vi "Chamber controller Dec 1 2016.vi"() -> ()   [LabVIEW 2014]
uses:
  <vilib>/Instr/_visa.llb/VISA Configure Serial Port (Instr).vi
  Environmental Chamber LabVIEW and Instruments/Drivers and Software/Keithley 2100 Series/Public/Configure/Configure 2 Wire Resistance.vi
  <vilib>/Utility/file.llb/Write To Spreadsheet File (string).vi
  <vilib>/Utility/file.llb/Read From Spreadsheet File (string).vi
  Environmental Chamber LabVIEW and Instruments/Drivers and Software/keithley_6430/Keithley 6430/Public/Data/Read (Single Point).vi
  Environmental Chamber LabVIEW and Instruments/Drivers and Software/LabVIEW 8.2 Drivers/keithley_24xx/Keithley 24XX/Public/Data/Read (Single Point).vi
  Environmental Chamber LabVIEW and Instruments/Drivers and Software/keithley_24xx/Keithley 24XX/Keithley 24XX.lvlib
  Environmental Chamber LabVIEW and Instruments/Drivers and Software/keithley_6430/Keithley 6430/Keithley 6430.lvlib
  Environmental Chamber LabVIEW and Instruments/Drivers and Software/Keithley 2100 Series/Keithley 2100 Series.lvlib
panel:
  in  "Arduino COMs":T1={"Arduino 1"="COM23", "Arduino 2"="COM24", "Arduino 3"="COM25", "Arduino 4"="COM26", "Arduino 5"="COM27", "Arduino 6"="COM28"}
  out "saving data?":bool
  out "ArduinoQCM\ncluster":T2 caption="Arduino QCM" {"6" format="%_8g"; "5" format="%_8g"; "4" format="%_8g"; "3" format="%_8g"; "2" format="%_8g"; "1" format="%#_10g"}
  in  "Data logging settings":T3={"Save during sequence only"=TRUE, "Save now"=FALSE, "sec between data points"=0.0, "Current data file path"=path "", "Save sample names"={"QCM1"="", "QCM2"="", "QCM3"="", "QCM4"="", "QCM5"="", "QCM6"="", "SRS"="", "K-2420"="", "K-6430"="", "K-2100"=""}, "Experiment Notes"=""} {"sec between data points" min=0.0 max=30.0 format="%#_13g"}
  in  "Sequence cluster":T4={"Save sequence"=FALSE, "Clear sequence"=FALSE, "Import sequence file"=FALSE, "Tare elapsed time"=TRUE, "Run Sequence"=FALSE, "Stop program when sequence ends"=TRUE, "User-defined\nsequence"=[], "Sequence end time"="", "Sequence\npreview"=[], "Current\nstep"=0, "Jump to next step"=FALSE} caption="Sequence settings"
  in  "Pressure parameters cluster":T5={"valve % open"=100.0, "Desired pressure"=0.0, "Vapor sccm"=0.0, "Gas sccm"=0.0, "Valve mode"=enum."% Open", "Pressure Mode"=enum."Abs. pressure", "analyte partial pressure"=23.8, "Turbo pump\nauto on"=TRUE, "Valve position (%)"=0.0, "read pressure"=0.0, "read vapor flow"=0.0, "read gas flow"=0.0, "pressure chart"={"pressure"=0.0}} caption="Pressure settings" {"read gas flow" format="%#_3g"; "read vapor flow" format="%#_3g"; "read pressure" format="%#_7f"; "Valve position (%)" format="%#_3g"; "analyte partial pressure" min=0.0 max=100.0 step=5.0; "Gas sccm" min=0 max=200 step=5; "Vapor sccm" min=0 max=200 step=5; "Desired pressure" min=0.0 max=760.0 step=5.0; "valve % open" min=0.0 max=100.0 step=5.0 format="%#_2f"}
  out "J-KEM temp chart":dbl(graph)
  out "Elapsed time (min)":dbl
  out "State date/time":string caption="Start time"
  out "K-2100 (Ohm)":cluster{"Measurement":dbl}(graph) caption="K-2100"
  out "K-6430":cluster{"Measurement":dbl}(graph)
  out "K-2420":cluster{"Resistance":sgl}(graph)
  in  "Gate time (sec)":enum16{"0.1", "1.0 ", "10"}(ring)=enum."1.0 "
  out "Hz":dbl format="%.7f"
  out "QCM plot":T6(graph)
  in  "Stop":bool
  in  "Clear all charts":bool
  out "O2 sensor output":dbl[](array[numeric]) caption="atm\nTorr"
  in  "rapidox O2 Sensor":bool
  in  "setnag O2 Pump":bool
  in  "Baud Rate 2":i32(ring)=2 items=["2400", "4800", "9600", "19200", "38400", "57600", "115200"]
  in  "Com Port":i32(ring) items=["Com 1", "Com 2", "Com 3", "Com 4", "Com 5", "Com 6", "COM 7", "COM 8", "COM 9", "COM 10", "COM 11", "COM 12", "com 13", "COM 14"]
  in  "Com Port 2":i32(ring) items=["Com 1", "Com 2", "Com 3", "Com 4", "Com 5", "Com 6", "COM 7", "COM 8", "COM 9", "COM 10", "COM 11", "COM 12", "com 13", "COM 14"]
  out "Waveform Chart":cluster{dbl}(graph)
  out "O2 Concentration (PPM)":dbl
  out "Waveform Chart 6":cluster{dbl}(graph)
  # "Currently Unused"
  # "100%"
  # "SRS"
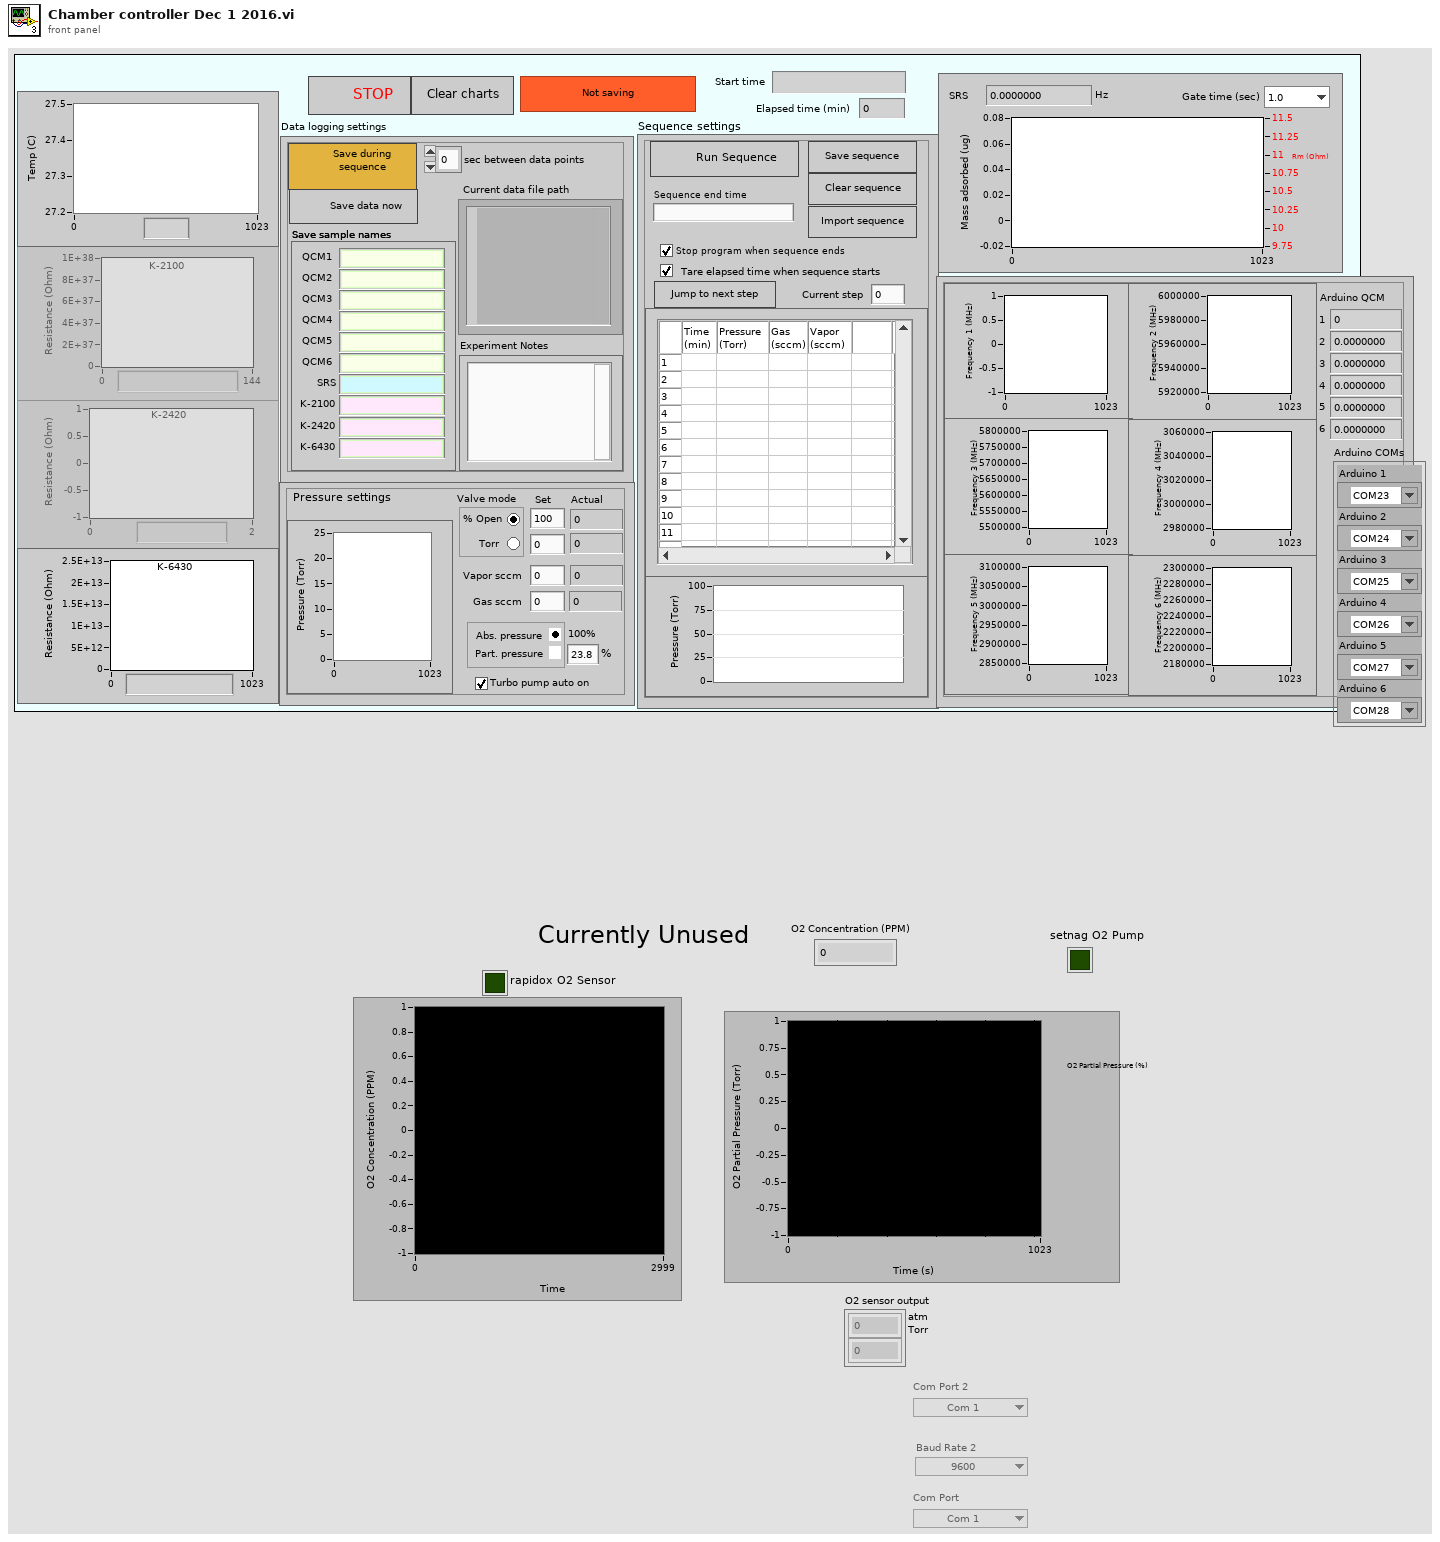
[diagram p1: front panel]
types:
  T1 = cluster{"Arduino 1":refnum<visa-resource-name>, "Arduino 2":refnum<visa-resource-name>, "Arduino 3":refnum<visa-resource-name>, "Arduino 4":refnum<visa-resource-name>, "Arduino 5":refnum<visa-resource-name>, "Arduino 6":refnum<visa-resource-name>}
  T2 = cluster{"arduino qcm 1":dbl, "1":dbl, "arduino qcm 2":dbl, "2":dbl, "arduino qcm 3":dbl, "3":dbl, "arduino qcm 4":dbl, "4":dbl, "arduino qcm 5":dbl, "5":dbl, "arduino qcm 6":dbl, "6":dbl}
  T3 = cluster{"Save during sequence only":bool, "Save now":bool, "sec between data points":dbl, "Current data file path":path, "Save sample names":cluster{"QCM1":string, "QCM2":string, "QCM3":string, "QCM4":string, "QCM5":string, "QCM6":string, "SRS":string, "K-2420":string, "K-6430":string, "K-2100":string}, "Experiment Notes":string}
  T4 = cluster{"Save sequence":bool, "Clear sequence":bool, "Import sequence file":bool, "Tare elapsed time":bool, "Run Sequence":bool, "Stop program when sequence ends":bool, "User-defined\nsequence":string[][], "Sequence end time":string, "Sequence\npreview":cluster{dbl[], dbl[]}[], "Current\nstep":i32, "Jump to next step":bool}
  T5 = cluster{"valve % open":dbl, "Desired pressure":dbl, "Vapor sccm":sgl, "Gas sccm":sgl, "Valve mode":enum32{"% Open", "Torr "}, "Pressure Mode":enum32{"Abs. pressure", " Part. pressure"}, "analyte partial pressure":dbl, "Turbo pump\nauto on":bool, "Valve position (%)":dbl, "read pressure":dbl, "read vapor flow":dbl, "read gas flow":dbl, "pressure chart":cluster{"pressure":dbl}}
  T6 = cluster{"Numeric Control":dbl, "Resistance out":dbl}
  T7 = cluster{"Keithley 6430":bool, "J-KEM":bool, "Keithley 2420":bool, "Keithley 2100":bool, "SRS QCM":bool, "Pressure control":bool, "Arduino":bool}
  T8 = enum8{"Enabled", "Disabled", "Disabled and Grayed Out"}
  T9 = enum16{"open", "open or create", "create or replace", "create", "open (read only)"}
  T10 = enum16{"no parity", "odd parity", "even parity", "mark parity", "space parity"}
  T11 = cluster{"String":string, "String":string, "String":string}
  T12 = cluster{"task out":refnum<k21>, "error out":errorcluster, "task out":refnum<k21>, "error out":errorcluster, "task out":refnum<k21>, "error out":errorcluster, "VISA resource name":refnum<visa-resource-name>, "error out":errorcluster}
  T13 = cluster{"task out":refnum<k21>, "error out":errorcluster, "task out":refnum<k21>, "error out":errorcluster, "task out":refnum<k21>, "error out":errorcluster, "VISA resource name out":refnum<visa-resource-name>, "error out":errorcluster}
  T14 = cluster{bool, "VISA resource name":refnum<visa-resource-name>, "error out":errorcluster}
  T15 = cluster{bool, "VISA resource name out":refnum<visa-resource-name>, "error out":errorcluster}
  T16 = cluster{"VISA resource name out":refnum<visa-resource-name>, "error out":errorcluster, "VISA resource name out":refnum<visa-resource-name>, "error out":errorcluster, "VISA resource name out":refnum<visa-resource-name>, "error out":errorcluster, "VISA resource name out":refnum<visa-resource-name>, "error out":errorcluster, "VISA resource name out":refnum<visa-resource-name>, "error out":errorcluster, "VISA resource name out 2":refnum<visa-resource-name>, "error out 2":errorcluster}
  T17 = cluster{bool, cluster{"task out":refnum<k21>, "error out":errorcluster, "task out":refnum<k21>, "error out":errorcluster, "task out":refnum<k21>, "error out":errorcluster, "VISA resource name out":refnum<visa-resource-name>, "error out":errorcluster}}
  T18 = cluster{"f":dbl, "f":dbl, "f":dbl, "f":dbl, "f":dbl, "f 2":dbl}
  T19 = cluster{"Boolean":bool, "VISA resource name out":refnum<visa-resource-name>, "error out":errorcluster}
  T20 = cluster{bool, "VISA out":refnum<visa-resource-name>, "error out":errorcluster}
  T21 = cluster{"Boolean":bool, "VISA out":refnum<visa-resource-name>, "error out":errorcluster}
  T22 = cluster{"Numeric Control":dbl, "Cluster":cluster{"Numeric Control":dbl}, "String":string, "error out":errorcluster}
  T23 = cluster{bool, "Com Port":i32, "Numeric Control out":dbl}
  T24 = cluster{"Arduino address":refnum<visa-resource-name>, "error in (no error)":errorcluster, "Arduino address 2":refnum<visa-resource-name>, "error in (no error) 2":errorcluster, "Arduino address 3":refnum<visa-resource-name>, "error in (no error) 3":errorcluster, "Arduino address 4":refnum<visa-resource-name>, "error in (no error) 4":errorcluster, "Arduino address 5":refnum<visa-resource-name>, "error in (no error) 5":errorcluster, "Arduino address 6":refnum<visa-resource-name>, "error in (no error) 6":errorcluster}
  T25 = cluster{"mean":string, "mean":string, "mean":string, "mean":string, "mean":string, "mean":string}
  T26 = cluster{"String data out":string, string, string, string}
  T27 = cluster{"valve % open":dbl, "Desired pressure":dbl, "Vapor sccm":sgl, "Gas sccm":sgl, "Valve mode":enum32{"% Open", "Torr "}, "Pressure Mode":enum32{"Abs. pressure", " Part. pressure"}, "analyte partial pressure":dbl, "Turbo pump\nauto on":bool}
  T28 = cluster{"User-defined\nsequence":string[][], "Present (s)":dbl, "current  step # in":i32, "sequence end time in":timestamp}
  T29 = cluster{"current  step # in":i32, "sequence end time in":timestamp, "Boolean":bool}
  T30 = cluster{"press/RH/gas/vapor":cluster{"pressure":string, "RH":string, "gas flow":string, "vapor flow":string}, "Cluster":cluster{"Valve position (%)":dbl, "read pressure":dbl, "read vapor flow":dbl, "read gas flow":dbl}}
  T31 = cluster{"Boolean":bool, "DAQ IDs in":cluster{"task out":refnum<k21>, "error out":errorcluster, "task out":refnum<k21>, "error out":errorcluster, "task out":refnum<k21>, "error out":errorcluster, "VISA Refnum out":refnum<visa-resource-name>, "error out":errorcluster}}
  T32 = cluster{"mean":dbl, "mean":dbl, "mean":dbl, "mean":dbl, "mean":dbl, "mean":dbl}
  T33 = cluster{"f":dbl, "f":dbl, "f":dbl, "f":dbl, "f":dbl}[]
  T34 = cluster{"pressure":string, "RH":string, "gas flow":string, "vapor flow":string}
  T35 = cluster{"Valve position (%)":dbl, "read pressure":dbl, "read vapor flow":dbl, "read gas flow":dbl}
  T36 = cluster{"mean":dbl, "mean":dbl, "mean":dbl, "mean":dbl, "mean":dbl, "mean":dbl, "mean":dbl, "mean":dbl, "mean":dbl, "mean":dbl, "mean":dbl, "mean":dbl}
  T37 = cluster{"QCM1":string, "QCM2":string, "QCM3":string, "QCM4":string, "QCM5":string, "QCM6":string, "SRS":string, "K-2420":string, "K-6430":string, "K-2100":string}
  T38 = cluster{"task out":refnum<k21>, "error out":errorcluster, "task out":refnum<k21>, "error out":errorcluster, "task out":refnum<k21>, "error out":errorcluster, "VISA Refnum out":refnum<visa-resource-name>, "error out":errorcluster}
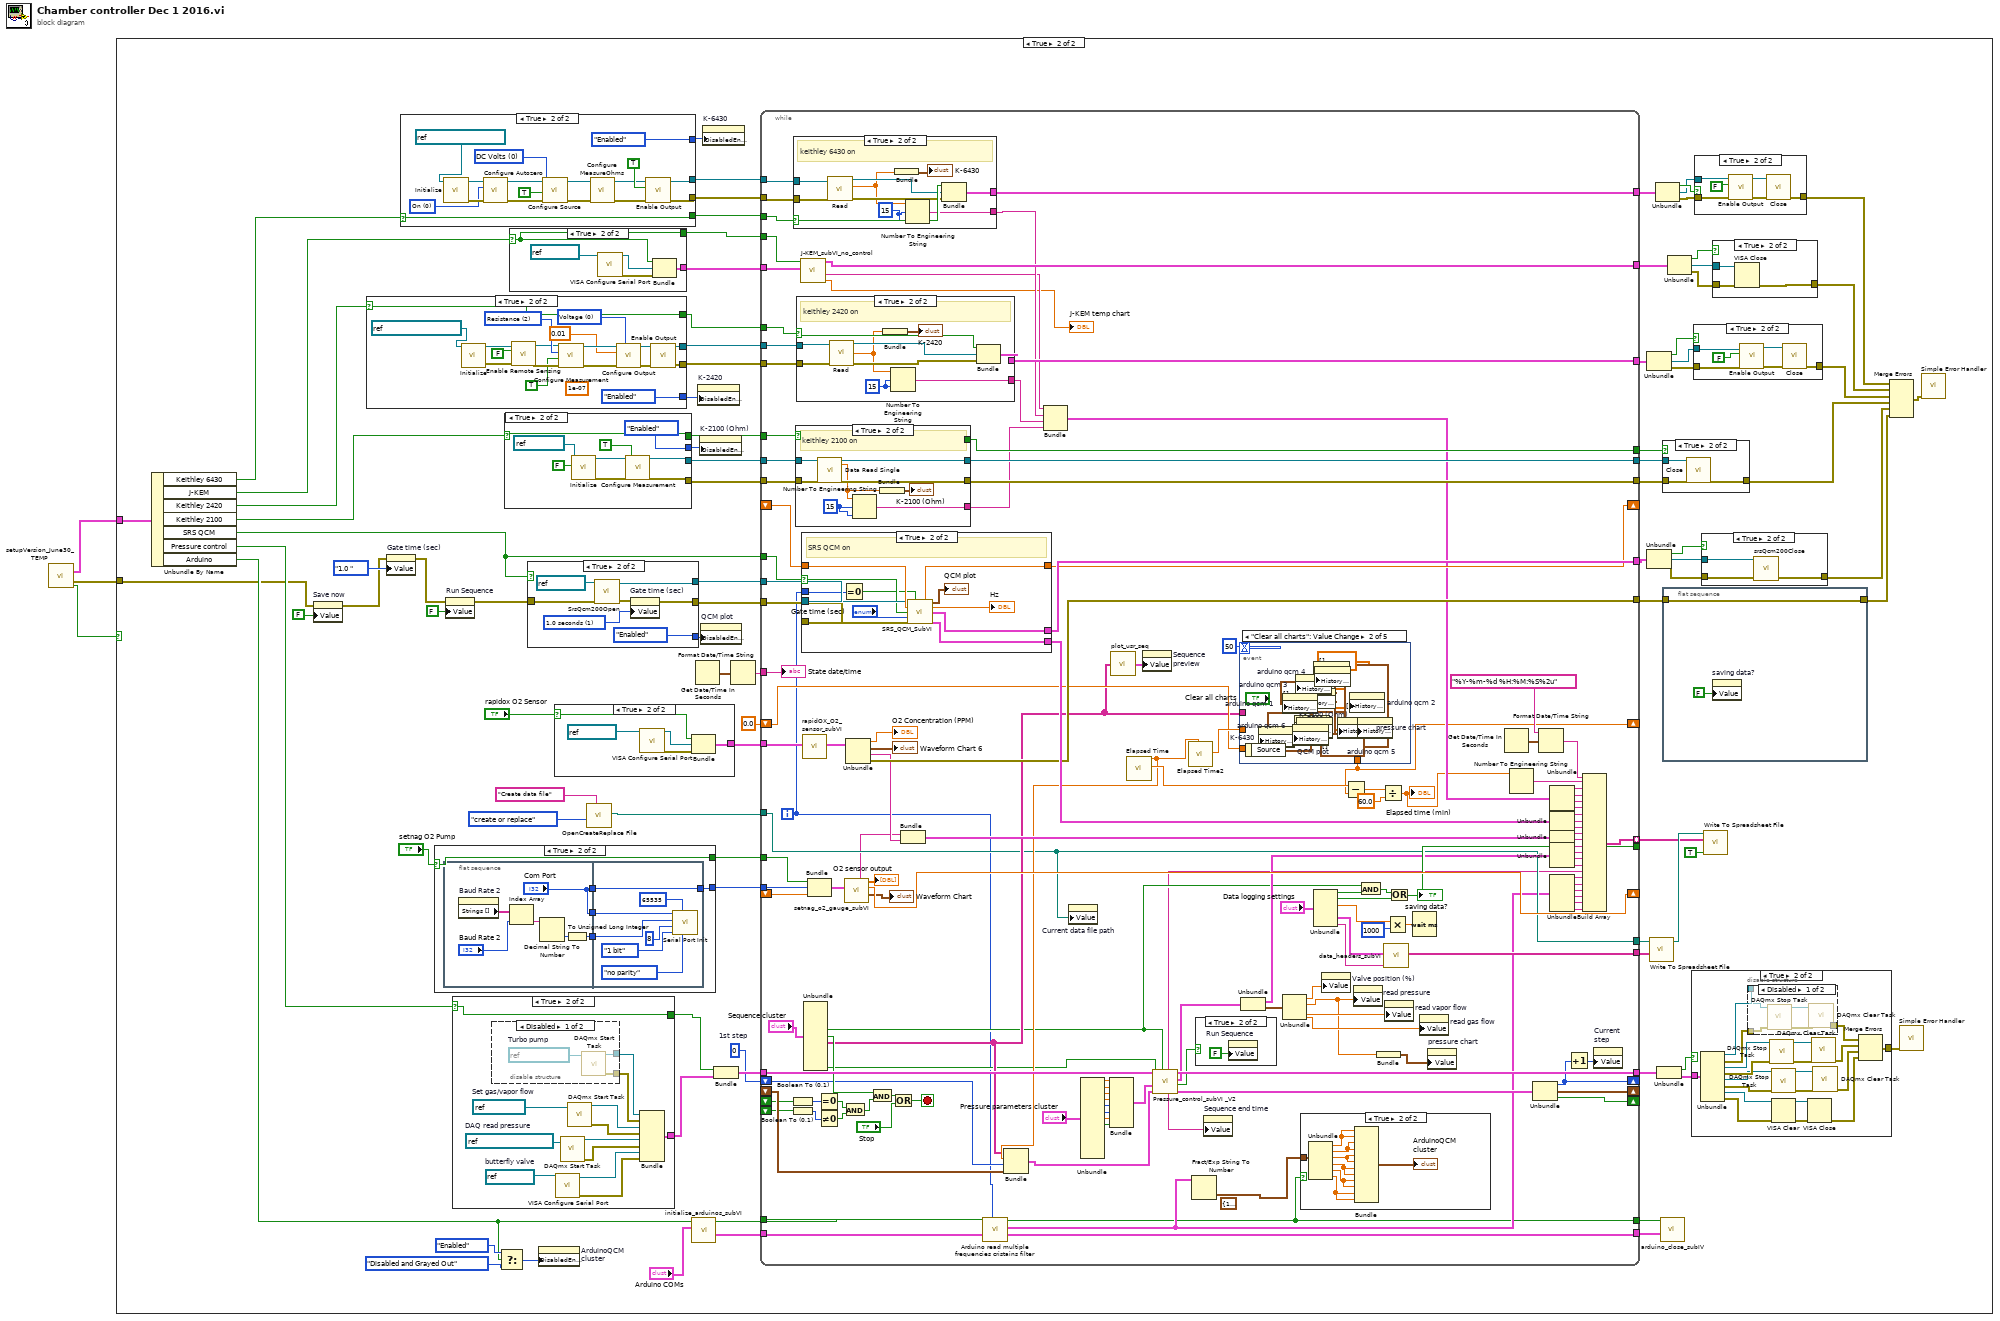
[diagram p0: block diagram]
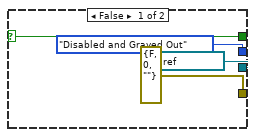
[diagram p4: hidden frame]
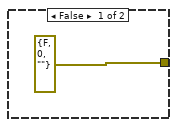
[diagram p5: hidden frame]
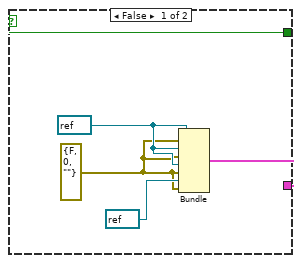
[diagram p7: hidden frame]
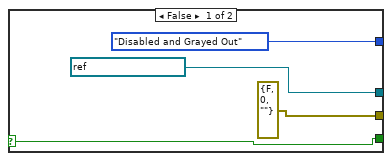
[diagram p10: hidden frame]
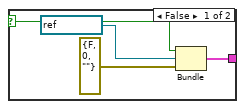
[diagram p11: hidden frame]
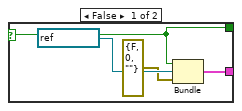
[diagram p13: hidden frame]
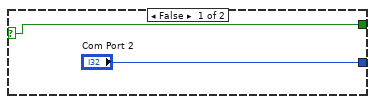
[diagram p14: hidden frame]
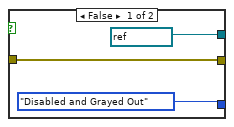
[diagram p16: hidden frame]
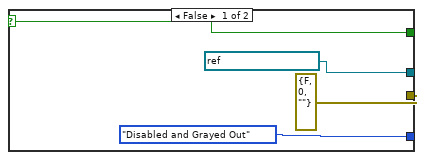
[diagram p18: hidden frame]
diagram:
  n1 = call "setupVersion_June30_TEMP.vi"() -> ("Instruments on/off"=w1:T7, "error IO"=w2:errorcluster, "OK"=w3:bool)  [unwired: 13 in]
  n2 = case shown="True" w3 {
    tunnel: w2 -> [_ w8]
    tunnel: w1 -> [_ w16]
    frame False {
    }
    frame True {
      w28 = 0  # 1st step
      n3 = Unbundle By Name(w16) -> ("Keithley 6430"=w15:bool, "J-KEM"=w14:bool, "Keithley 2420"=w13:bool, "Keithley 2100"=w12:bool, "SRS QCM"=w11:bool, "Pressure control"=w10:bool, "Arduino"=w9:bool)
      n4 = property on="Save now" class="Bool (strict)"(error in=w8, "Value"=FALSE) -> (error out=w7:errorcluster)  [unwired: 1 in, 1 out]
      n5 = case shown="True" w13 {
        selector: w13 -> [w252 w256]
        tunnel: [refnum<visa-resource-name> "GPIB1::24::INSTR" ("VISA resource name") w265] -> w92
        tunnel: [errorcluster {"status"=FALSE, "code"=0, "source"=""} ("error out") w260] -> w91
        tunnel: [T8."Disabled and Grayed Out" ("Disabled") T8."Enabled" ("Disabled")] -> w55
        tunnel: [w252 w256] -> w48
        frame False {
        }
        frame True {
          (unwired) 1e-07 ("Manual Range (1.0)")
          w267 = u16 0 items=["Voltage", "Current"] ("Source Mode  (0: Voltage)")
          w272 = u16 2 items=["Volts", "Current", "Resistance"] ("Function (0: Volts)")
          n6 = call "Initialize.vi"("VISA resource name"=refnum<visa-resource-name> "GPIB1::24::INSTR") -> ("error out"=w261:errorcluster, "VISA resource name out"=w264:refnum<visa-resource-name>)  [unwired: 9 in]
          n7 = call "Enable Remote Sensing.vi"("error in (no error)"=w261, "Enable Remote Sensing (T: Enable)"=FALSE ("4-wire?"), "VISA resource name"=w264) -> ("error out"=w262:errorcluster, "VISA resource name out"=w263:refnum<visa-resource-name>)  [unwired: 7 in]
          n8 = call "Configure Measurement.vi"("error in (no error)"=w262, "Enable Auto Range (T:Enable)"=TRUE, "Function (0: Volts)"=w272, "VISA resource name"=w263) -> ("error out"=w271:errorcluster, "VISA resource name out"=w270:refnum<visa-resource-name>)  [unwired: 6 in]
          n9 = call "Configure Output.vi"("Source Mode  (0: Voltage)"=w267, "error in (no error)"=w271, "Output Level (0)"=0.01 ("Applied Voltage (V)"), "VISA resource name"=w270) -> ("error out"=w269:errorcluster, "VISA resource name out"=w268:refnum<visa-resource-name>)  [unwired: 6 in]
          n10 = call "Enable Output.vi"("error in (no error)"=w269, "VISA resource name"=w268) -> ("error out"=w260:errorcluster, "VISA resource name out"=w265:refnum<visa-resource-name>)  [unwired: 8 in]
        }
      }
      n11 = property on="Gate time (sec)" class="Enum (strict)"(error in=w7, "Value"=enum16{"0.1", "1.0 ", "10"}."1.0 " ("Gate time (sec)")) -> (error out=w17:errorcluster)  [unwired: 1 in, 1 out]
      n12 = case shown="True" w15 {
        selector: w15 -> [w168 w172]
        tunnel: [refnum<visa-resource-name> "GPIB0::29::INSTR" ("VISA resource name") w183] -> w61
        tunnel: [errorcluster {"status"=FALSE, "code"=0, "source"=""} ("error out") w184] -> w60
        tunnel: [T8."Disabled and Grayed Out" ("Disabled") T8."Enabled" ("Disabled")] -> w54
        tunnel: [w168 w172] -> w47
        frame False {
        }
        frame True {
          w173 = u16 0 items=["DC Volts", "DC Current"] ("Source Function (0: DC Volts)")
          w180 = u16 0 items=["On", "Off", "Once"] ("Autozero  (0: On)")
          n13 = call "Initialize.vi"("VISA resource name"=refnum<visa-resource-name> "GPIB0::29::INSTR") -> ("error out"=w181:errorcluster, "VISA resource name out"=w182:refnum<visa-resource-name>)  [unwired: 4 in, 5 out]
          n14 = call "Configure Autozero.vi"("error in (no error)"=w181, "Autozero  (0: On)"=w180, "VISA resource name"=w182) -> ("error out"=w176:errorcluster, "VISA resource name out"=w178:refnum<visa-resource-name>)  [unwired: 7 in]
          n15 = call "Configure Source.vi"("error in (no error)"=w176, "Auto Range (T:Enable)"=TRUE, "Source Function (0: DC Volts)"=w173, "VISA resource name"=w178) -> ("error out"=w175:errorcluster, "VISA resource name out"=w177:refnum<visa-resource-name>)  [unwired: 6 in]
          n16 = call "Configure MeasureOhms.vi"("error in (no error)"=w175, "VISA resource name"=w177) -> ("error out"=w188:errorcluster, "VISA resource name out"=w186:refnum<visa-resource-name>)  [unwired: 4 in, 4 out]
          n17 = call "Enable Output.vi"("error in (no error)"=w188, "Enable Output (F:Off)"=TRUE ("Output (F:Off)"), "VISA resource name"=w186) -> ("error out"=w184:errorcluster, "VISA resource name out"=w183:refnum<visa-resource-name>)  [unwired: 7 out]
        }
      }
      n18 = case shown="True" "setnag O2 Pump" {
        selector: "setnag O2 Pump" -> [w211 w213]
        tunnel: ["Com Port 2" w214] -> w88
        tunnel: [w211 w213] -> w36
        frame False {
        }
        frame True {
          n19 = flat-sequence {
            tunnel: ["Com Port"] -> w217
            tunnel: [w219] -> w216
            tunnel: ["Com Port"] -> w215
            tunnel: w217 -> [w225]
            tunnel: w216 -> [w224]
            tunnel: w215 -> [w226]
            tunnel: [w226] -> w214
            frame #0 {
              n20 = property on="Baud Rate 2" class="Ring (strict)"() -> ("Strings []"=w221:string[])  [unwired: 2 in, 2 out]
              n21 = Index Array(array=w221, index="Baud Rate 2") -> (element=w222:string)
              n22 = Decimal String To Number(string=w222) -> (number=w220:i32)  [unwired: 2 in, 1 out]
              n23 = To Unsigned Long Integer(number=w220) -> (unsigned 32bit integer=w219:u32)
            }
            frame #1 {
              n24 = call <vilib>:"Serial Port Init.vi"("parity"=T10."no parity", "buffer size"=u16 65535, "stop bits"=enum16{"1 bit", "1.5 bits", "2 bits"}."1 bit", "data bits"=u16 8, "baud rate"=w224, "port number"=w225) -> ()  [unwired: 1 in, 1 out]
            }
          }
        }
      }
      n25 = property on="Run Sequence" class="Bool (strict)"(error in=w17, "Value"=FALSE) -> (error out=w23:errorcluster)  [unwired: 1 in, 1 out]
      n26 = case shown="True" w10 {
        selector: w10 -> [w140 w145]
        tunnel: [w141 w147] -> w30
        tunnel: [w140 w145] -> w31
        frame False {
          w143 = refnum<k21> refnum ("task out")
          w142 = errorcluster {"status"=FALSE, "code"=0, "source"=""} ("error out")
          n27 = Bundle("task out"=w143, "error out"=w142, "task out"=w143, "error out"=w142, "task out"=w143, "error out"=w142, "VISA resource name"=refnum<visa-resource-name> refnum, "error out"=w142) -> (w141:T12)  [unwired: 1 in]
        }
        frame True {
          w155 = refnum<visa-resource-name> "COM5"  # butterfly valve
          w156 = refnum<k21> "Setflow"  # Set gas/vapor flow
          w157 = refnum<k21> "AllDaqReadings"  # DAQ read pressure
          n28 = disable-structure shown="Disabled" {
            disable-tunnel: [w159 _] -> w154
            disable-tunnel: [w158 _] -> w153
            frame Disabled {
              w160 = refnum<k21> "TurboON"  # Turbo pump
              n29 = call <vilib>:"DAQmx Start Task.vi"("task/channels in"=w160) -> ("task out"=w159:refnum<k21>, "error out"=w158:errorcluster)  [unwired: 13 in]
            }
            frame Enabled {
            }
          }
          n30 = call-poly "VISA Configure Serial Port"("VISA resource name"=w155) -> ("VISA resource name out"=w148:refnum<visa-resource-name>, "error out"=w146:errorcluster)  [unwired: 13 in]
          n31 = call <vilib>:"DAQmx Start Task.vi"("task/channels in"=w157) -> ("task out"=w150:refnum<k21>, "error out"=w149:errorcluster)  [unwired: 13 in]
          n32 = call <vilib>:"DAQmx Start Task.vi"("task/channels in"=w156) -> ("task out"=w152:refnum<k21>, "error out"=w151:errorcluster)  [unwired: 13 in]
          n33 = Bundle("task out"=w154, "error out"=w153, "task out"=w152, "error out"=w151, "task out"=w150, "error out"=w149, "VISA resource name out"=w148, "error out"=w146) -> (w147:T13)  [unwired: 1 in]
        }
      }
      n34 = Select(t=T8."Enabled" ("Disabled"), s=w9, f=T8."Disabled and Grayed Out" ("Disabled")) -> (s? t:f=w22:T8)
      n35 = case shown="True" w12 {
        selector: w12 -> [w102 w107]
        tunnel: [refnum<visa-resource-name> "K-2100" ("VISA resource name out") w110] -> w45
        tunnel: [errorcluster {"status"=FALSE, "code"=0, "source"=""} ("error out") w109] -> w44
        tunnel: [w102 w107] -> w43
        tunnel: [T8."Disabled and Grayed Out" ("Disabled") T8."Enabled" ("Disabled")] -> w38
        frame False {
        }
        frame True {
          n36 = call "Initialize.vi"("VISA resource name"=refnum<visa-resource-name> "K-2100", "Reset? (T: Reset)"=FALSE) -> ("VISA resource name out"=w111:refnum<visa-resource-name>, "error out"=w108:errorcluster)  [unwired: 16 in]
          n37 = call-poly "Configure Measurement.vi"("VISA resource name"=w111, "error in (no error)"=w108, "Auto Range? (T: Auto)"=TRUE) -> ("VISA resource name out"=w110:refnum<visa-resource-name>, "error out"=w109:errorcluster)  [unwired: 15 in]
        }
      }
      n38 = case shown="True" w14 {
        selector: w14 -> [w202 w207]
        tunnel: [w203 w208] -> w77
        tunnel: [w202 w207] -> w71
        frame False {
          n39 = Bundle(w202, "VISA resource name"=refnum<visa-resource-name> "COM3", "error out"=errorcluster {"status"=FALSE, "code"=0, "source"=""}) -> (w203:T14)  [unwired: 1 in]
        }
        frame True {
          n40 = call-poly "VISA Configure Serial Port"("VISA resource name"=refnum<visa-resource-name> "COM3") -> ("VISA resource name out"=w209:refnum<visa-resource-name>, "error out"=w206:errorcluster)  [unwired: 13 in]
          n41 = Bundle(w207, "VISA resource name out"=w209, "error out"=w206) -> (w208:T15)  [unwired: 1 in]
        }
      }
      n42 = case shown="True" w11 {
        tunnel: [refnum<visa-resource-name> "COM6" ("VISA in") w241] -> w90
        tunnel: [w236 w238] -> w89
        tunnel: w23 -> [w236 w243]
        tunnel: [T8."Disabled and Grayed Out" ("Disabled") T8."Enabled" ("Disabled")] -> w56
        frame False {
        }
        frame True {
          w240 = u16 1 items=["0.1 seconds", "1.0 seconds", "10.0 seconds"] ("Gate time")
          n43 = call "SrsQcm200Open.vi"("error in"=w243, "VISA in"=refnum<visa-resource-name> "COM6") -> ("error out"=w239:errorcluster, "VISA out"=w241:refnum<visa-resource-name>)  [unwired: 3 in]
          n44 = property on="Gate time (sec)" class="Enum (strict)"(error in=w239, "Value"=w240) -> (error out=w238:errorcluster)  [unwired: 1 in, 1 out]
        }
      }
      n45 = property on="ArduinoQCM\ncluster" class="Clust (strict)"("DisabledEnum"=w22) -> ()  [unwired: 2 in, 2 out]
      n46 = case shown="True" "rapidox O2 Sensor" {
        selector: "rapidox O2 Sensor" -> [w189 w194]
        tunnel: [w190 w195] -> w67
        frame False {
          n47 = Bundle(w189, "VISA resource name"=refnum<visa-resource-name> "COM7", "error out"=errorcluster {"status"=FALSE, "code"=0, "source"=""}) -> (w190:T14)  [unwired: 1 in]
        }
        frame True {
          n48 = call-poly "VISA Configure Serial Port"("VISA resource name"=refnum<visa-resource-name> "COM7") -> ("VISA resource name out"=w196:refnum<visa-resource-name>, "error out"=w193:errorcluster)  [unwired: 13 in]
          n49 = Bundle(w194, "VISA resource name out"=w196, "error out"=w193) -> (w195:T15)  [unwired: 1 in]
        }
      }
      n50 = call "OpenCreateReplace File.vi"("prompt"="Create data file", "function (open:0)"=T9."create or replace") -> ("new file path"=w46:path)  [unwired: 6 in, 3 out]
      n51 = call "initialize_arduinos_subVI.vi"("arduino 1-6 addresses"="Arduino COMs", "arduinos on?"=w9) -> ("arduino addresses/errors"=w32:T16, "arduinos on/off"=w52:bool)  [unwired: 8 in]
      n52 = Get Date/Time In Seconds() -> (seconds since 1Jan1904=w94:timestamp)
      n53 = property on="K-2420" class="WFChart (strict)"("DisabledEnum"=w55) -> ()  [unwired: 2 in, 2 out]
      n54 = property on="K-2100 (Ohm)" class="WFChart (strict)"("DisabledEnum"=w38) -> ()  [unwired: 2 in, 2 out]
      n55 = property on="QCM plot" class="WFChart (strict)"("DisabledEnum"=w56) -> ()  [unwired: 2 in, 2 out]
      n56 = property on="K-6430" class="WFChart (strict)"("DisabledEnum"=w54) -> ()  [unwired: 2 in, 2 out]
      n57 = Bundle(w31, w30) -> (w29:T17)  [unwired: 1 in]
      n58 = Format Date/Time String(seconds (now)=w94) -> (date/time string=w35:string)  [unwired: 2 in]
      n59 = while {
        shift-right: [w417] -> _
        shift-left: _ -> [w348]
        tunnel: [w401] -> w53 mode=indexing if=w370
        tunnel: w48 -> [w406]
        tunnel: w92 -> [w416]
        tunnel: w91 -> [w415]
        tunnel: w90 -> [w414]
        tunnel: w89 -> [w413]
        tunnel: w11 -> [w412]
        tunnel: w36 -> [w350]
        tunnel: w88 -> [w351]
        tunnel: [w411] -> w85
        tunnel: [w410] -> w81
        tunnel: w77 -> [w409]
        tunnel: [w408] -> w76
        tunnel: w71 -> [w407]
        tunnel: w67 -> [w359]
        tunnel: [w355] -> w5
        tunnel: [w290] -> w66
        tunnel: w46 -> [w290]
        shift-right: [w399] -> _
        shift-left: _ -> [w400]
        tunnel: w61 -> [w405]
        tunnel: w60 -> [w404]
        tunnel: [w403] -> w59
        tunnel: [w370] -> _
        tunnel: w52 -> [w277]
        tunnel: w32 -> [w280]
        tunnel: [w276] -> w50
        tunnel: [w278] -> w51
        tunnel: [w387] -> w49
        tunnel: w47 -> [w382]
        tunnel: w45 -> [w369]
        tunnel: w44 -> [w368]
        tunnel: w43 -> [w367]
        tunnel: [w366] -> w42
        tunnel: [w365] -> w41
        tunnel: [w364] -> w40
        shift-right: [w342] -> _
        shift-left: 0.0 ("Elapsed Time (s)") -> [w343]
        tunnel: w35 -> [w333]
        tunnel: w29 -> [w315]
        shift-right: [w285] -> _
        shift-left: w28 -> [w304]
        shift-right: [w310] -> _
        shift-left: _ -> [w308]
        shift-right: [w309] -> _
        shift-left: _ -> [w307]
        shift-left: _ -> [w306]
        tunnel: [w302] -> w27
        i -> [w275]
        stop <- w372 stop-if-true
        (unwired) T18 {"f"=1000000.0, "f"=1000000.0, "f"=1000000.0, "f"=1000000.0, "f"=1000000.0, "f 2"=1000000.0} ("y")
        n60 = Boolean To (0,1)(Boolean=w307) -> (0, 1=w380:i16)
        n61 = Boolean To (0,1)(Boolean=w306) -> (0, 1=w379:i16)
        n62 = case "Keithley 6430" shown="True" w382 {
          selector: w382 -> [w452 w463]
          tunnel: w405 -> [w451 w460]
          tunnel: w404 -> [w450 w459]
          tunnel: ["" w462] -> w354
          tunnel: [w449 w461] -> w403
          frame False {
            # "keithley 6430 off"
            n63 = Bundle(w452, "VISA resource name out"=w451, "error out"=w450) -> (w449:T15)  [unwired: 1 in]
          }
          frame True {
            w454 = i16 15 ("width (-)")
            # "keithley 6430 on"
            n64 = call-poly "Read.vi"("error in (no error)"=w459, "VISA resource name"=w460) -> ("error out"=w458:errorcluster, "Measurement"=w456:dbl, "VISA resource name out"=w457:refnum<visa-resource-name>)  [unwired: 1 in, 6 out]
            n65 = Bundle("Measurement"=w456) -> (→"K-6430":cluster{"Measurement":dbl})  [unwired: 1 in]
            n66 = Number To Engineering String(2:w454, 3:w454, 4:w456) -> (0:w462:string)  [unwired: 1 in]
            n67 = Bundle(w463, "VISA resource name out"=w457, "error out"=w458) -> (w461:T15)  [unwired: 1 in]
          }
        }
        n68 = case shown="True" w367 {
          selector: w367 -> [w428 w433]
          tunnel: [w429 w440] -> w365
          tunnel: [w430 w439] -> w364
          tunnel: w369 -> [w429 w438]
          tunnel: w368 -> [w430 w437]
          tunnel: ["" w435] -> w352
          tunnel: [w428 w433] -> w366
          frame False {
            # "keithley 2100 off"
          }
          frame True {
            w432 = i16 15 ("width (-)")
            # "keithley 2100 on"
            n69 = call "Data Read Single.vi"("VISA resource name"=w438, "error in (no error)"=w437) -> ("VISA resource name out"=w440:refnum<visa-resource-name>, "Measurement"=w436:dbl, "error out"=w439:errorcluster)  [unwired: 15 in]
            n70 = Number To Engineering String ("elapsed time (min)")(2:w432, 3:w432, 4:w436) -> (0:w435:string)  [unwired: 1 in]
            n71 = Bundle("Measurement"=w436) -> (→"K-2100 (Ohm)":cluster{"Measurement":dbl})  [unwired: 1 in]
          }
        }
        n72 = case "Keithley 2420" shown="True" w406 {
          selector: w406 -> [w467 w476]
          tunnel: w416 -> [w466 w471]
          tunnel: w415 -> [w465 w470]
          tunnel: [w464 w474] -> w411
          tunnel: ["" w473] -> w353
          frame False {
            # "keithley 2420 off"
            n73 = Bundle(w467, "VISA resource name out"=w466, "error out"=w465) -> (w464:T15)  [unwired: 1 in]
          }
          frame True {
            w469 = i16 15 ("width (-)")
            # "keithley 2420 on"
            n74 = call-poly "Read.vi"("VISA resource name"=w471, "error in (no error)"=w470) -> ("VISA resource name out"=w477:refnum<visa-resource-name>, "Resistance"=w472:sgl, "error out"=w475:errorcluster)  [unwired: 7 in, 4 out]
            n75 = Bundle("Resistance"=w472) -> (→"K-2420":cluster{"Resistance":sgl})  [unwired: 1 in]
            n76 = Number To Engineering String(2:w469, 3:w469, 4:w472) -> (0:w473:string)  [unwired: 1 in]
            n77 = Bundle(w476, "VISA resource name out"=w477, "error out"=w475) -> (w474:T15)  [unwired: 1 in]
          }
        }
        n78 = call "J-KEM_subVI_no_control.vi"("Address in"=w409, "J-KEM on?"=w407) -> ("Temp (C)"=→"J-KEM temp chart":dbl, "String data out"=w341:string, "Address out"=w408:T19)  [unwired: 6 in, 1 out]
        n79 = case "SRS QCM" shown="True" w412 {
          selector: w412 -> [w481 w490]
          tunnel: w414 -> [w484 w492]
          tunnel: w413 -> [w483 w493]
          tunnel: [w482 w496] -> w410
          tunnel: w400 -> [w479 w495]
          tunnel: [w479 w494] -> w399
          tunnel: [T11 {"String"="", "String"="", "String"=""} ("M,F,MR output cluster") w489] -> w392
          tunnel: w275 -> [_ w486]
          frame False {
            # "SRS QCM off"
            n80 = Bundle(w481, "VISA out"=w484, "error out"=w483) -> (w482:T20)  [unwired: 1 in]
          }
          frame True {
            # "SRS QCM on"
            n81 = Equal To 0?(x=w486) -> (x = 0?=w487:bool)
            n82 = call "SRS_QCM_SubVI.vi"("VISA Refnum in"=w492, "first iteration?"=w487, "Frequency out 3"=w495, "Boolean 2"=w490, "Gate time"="Gate time (sec)", "error in (no error)"=w493) -> ("Frequency out 2"=w494:dbl, "Cluster"=→"QCM plot":T6, "Frequency out"=→"Hz":dbl, "Cluster 2"=w496:T21, "M,F,MR output cluster"=w489:T11)  [unwired: 2 in, 3 out]
          }
        }
        n83 = call "rapidOX_O2_sensor_subVI.vi"("rapid ox info in"=w359) -> ("rapidox info out"=w358:T22)  [unwired: 10 in]
        n84 = Unbundle("Sequence cluster") -> ("Run Sequence"=w296:bool, "Stop program when sequence ends"=w305:bool, "User-defined\nsequence"=w300:string[][], "Jump to next step"=w286:bool)  [unwired: 7 out]
        n85 = Bundle(w350, "Com Port"=w351, "Numeric Control out"=w348) -> (w349:T23)  [unwired: 1 in]
        n86 = Equal To 0?(x=w380) -> (x = 0?=w377:bool)
        n87 = Not Equal To 0?(x=w379) -> (x != 0?=w378:bool)
        n88 = And(x=w377, y=w378) -> (x .and. y?=w371:bool)
        n89 = call "setnag_o2_gauge_subVI.vi"("setnag info in"=w349) -> ("Cluster"=→"Waveform Chart":cluster{"Numeric Control":dbl}, "Numeric Control out"=w417:dbl, "Array"=→"O2 sensor output":dbl[], "String"=w287:string)  [unwired: 7 in]
        n90 = Unbundle(w358) -> ("Numeric Control"=→"O2 Concentration (PPM)":dbl, "Cluster"=→"Waveform Chart 6":cluster{"Numeric Control":dbl}, "String"=w332:string, "error out"=w355:errorcluster)
        n91 = And(x=w305, y=w371) -> (x .and. y?=w346:bool)
        n92 = Or(x=w346, y="Stop") -> (x .or. y?=w372:bool)
        n93 = Bundle("String"=w287, "String"=w332) -> (w331:cluster{"String":string, "String":string})  [unwired: 1 in]
        n94 = call "Arduino read multiple frequencies cristains filter.vi"("main loop iteration number"=w275, "arduino addresses in"=w280, "arduinos on?"=w277) -> ("arduino addresses out"=w278:T24, "arduino frequencies out"=w279:T25, "arduinos on"=w276:bool)  [unwired: 6 in]
        n95 = Bundle("String data out"=w341, w354, w353, w352) -> (w347:T26)  [unwired: 1 in]
        n96 = property on="Current data file path" class="Path"("Value"=w290) -> ()  [unwired: 2 in, 2 out]
        n97 = Unbundle("Pressure parameters cluster") -> ("valve % open"=w320:dbl, "Desired pressure"=w322:dbl, "Vapor sccm"=w323:sgl, "Gas sccm"=w324:sgl, "Valve mode"=w325:enum32{"% Open", "Torr "}, "Pressure Mode"=w326:enum32{"Abs. pressure", " Part. pressure"}, "analyte partial pressure"=w327:dbl, "Turbo pump\nauto on"=w328:bool)  [unwired: 5 out]
        n98 = Bundle("valve % open"=w320, "Desired pressure"=w322, "Vapor sccm"=w323, "Gas sccm"=w324, "Valve mode"=w325, "Pressure Mode"=w326, "analyte partial pressure"=w327, "Turbo pump\nauto on"=w328) -> (w319:T27)  [unwired: 1 in]
        n99 = call "plot_usr_seq.vi"("User-defined sequence"=w300) -> ("Sequence Preview"=w292:cluster{dbl[], dbl[]}[])
        n100 = call "Elapsed Time"() -> ("Present (s)"=w312:dbl, "Elapsed Time (s)"=w361:dbl)  [unwired: 12 in, 6 out]
        n101 = Bundle("User-defined\nsequence"=w300, "Present (s)"=w312, "current  step # in"=w304, "sequence end time in"=w308) -> (w313:T28)  [unwired: 1 in]
        n102 = property on="Sequence\npreview" class="XYGraph (strict)"("Value"=w292) -> ()  [unwired: 2 in, 2 out]
        n103 = call "Pressure_control_subVI _V2.vi"("Run Sequence"=w296, "user sequence, present (s) in, current step in, seq time in"=w313, "pressure parameters in"=w319, "Jump to next step"=w286, "pressure control on? / DAQ IDs/errors in"=w315) -> ("current step # out, shift register time out, seq button on?"=w311:T29, "sequence over? USE THIS TO REINITIALIZE RUN SEQUENCE BUTTON SO PROGRAM ENDS"=w301:bool, "save press/RH/gasflow/vaporflow - read valve position/pressure/vaporflow/gasflow"=w299:T30, "pressure control on out, DAQ IDs/errors out"=w302:T31, "sequence end date/time string"=w303:string, "pressure_setpoint"=w282:string)  [unwired: 1 in]
        n104 = call "Elapsed Time2"("Set Start Time (s)"=w312) -> ("Elapsed Time (s)"=w344:dbl)  [unwired: 11 in, 7 out]
        n105 = Fract/Exp String To Number(string=w279) -> (number=w274:T32)  [unwired: 3 in, 1 out]
        n106 = case shown="True" w301 {
          frame False {
          }
          frame True {
            n107 = property on="Run Sequence" class="Bool (strict)"("Value"=FALSE ("Run Sequence")) -> ()  [unwired: 2 in, 2 out]
          }
        }
        n108 = property on="Sequence end time" class="Str"("Value"=w303) -> ()  [unwired: 2 in, 2 out]
        n109 = event shown="[1] \"Clear all charts\": Value Change" {
          selector: _ -> [_ _ _ _ _]
          dyn-events: _ -> [_ _ _ _ _]
          timeout: 50 -> [_ _ _ _ _]
          tunnel: w300 -> [_ _ _ w447 _]
          tunnel: w344 -> [_ _ _ _ _]
          tunnel: w343 -> [w441 _ _ _ _]
          tunnel: [w441 _ _ _ _] -> w342
          event Timeout {
            n110 = event-data() -> ()  [unwired: 1 in, 1 out]
          }
          event "Clear all charts": Value Change {
            (unwired) T33 [] ("History Data")
            w444 = cluster{dbl}[] [] ("History Data")
            w445 = cluster{"Resistance":sgl}[] [] ("History Data")
            w442 = dbl[] [] ("History Data")
            n111 = event-data() -> ()  [unwired: 1 in, 1 out]
            n112 = property on="K-6430" class="WFChart (strict)"("History Data"=w445) -> ()  [unwired: 2 in, 2 out]
            n113 = property on="arduino qcm 1" class="WFChart (strict)"("History Data"=w442) -> ()  [unwired: 2 in, 2 out]
            n114 = property on="Waveform Chart" class="WFChart (strict)"("History Data"=w444) -> ()  [unwired: 2 in, 2 out]
            n115 = property on="arduino qcm 6" class="WFChart (strict)"("History Data"=w442) -> ()  [unwired: 2 in, 2 out]
            n116 = property on="arduino qcm 3" class="WFChart (strict)"("History Data"=w442) -> ()  [unwired: 2 in, 2 out]
            n117 = property on="QCM plot" class="WFChart (strict)"("History Data"=cluster{dbl, "Resistance out":dbl}[] []) -> ()  [unwired: 2 in, 2 out]
            n118 = property on="K-2100 (Ohm)" class="WFChart (strict)"("History Data"=w445) -> ()  [unwired: 2 in, 2 out]
            n119 = property on="arduino qcm 4" class="WFChart (strict)"("History Data"=w442) -> ()  [unwired: 2 in, 2 out]
            n120 = property on="K-2420" class="WFChart (strict)"("History Data"=w445) -> ()  [unwired: 2 in, 2 out]
            n121 = property on="pressure chart" class="WFChart (strict)"("History Data"=w444) -> ()  [unwired: 2 in, 2 out]
            n122 = property on="arduino qcm 2" class="WFChart (strict)"("History Data"=w442) -> ()  [unwired: 2 in, 2 out]
            n123 = property on="arduino qcm 5" class="WFChart (strict)"("History Data"=w442) -> ()  [unwired: 2 in, 2 out]
          }
          event "Sequence cluster.Clear sequence": Value Change {
            n124 = event-data() -> ()  [unwired: 1 in, 1 out]
            n125 = property on="User-defined\nsequence" class="Tbl (strict)"("Value"=string[][] []) -> ()  [unwired: 2 in, 2 out]
          }
          event "Sequence cluster.Save sequence": Value Change {
            n126 = event-data() -> ()  [unwired: 1 in, 1 out]
            n127 = call-poly <vilib>:"Write To Spreadsheet File.vi"("2D data"=w447) -> ()  [unwired: 7 in, 1 out]
          }
          event "Sequence cluster.Import sequence file": Value Change {
            n128 = event-data() -> ()  [unwired: 1 in, 1 out]
            n129 = call-poly <vilib>:"Read From Spreadsheet File.vi"() -> ("all rows"=w448:string[][])  [unwired: 7 in, 4 out]
            n130 = property on="User-defined\nsequence" class="Tbl (strict)"("Value"=w448) -> ()  [unwired: 2 in, 2 out]
          }
        }
        n131 = Unbundle(w299) -> ("press/RH/gas/vapor"=w298:T34, "Cluster"=w297:T35)
        n132 = Unbundle(w297) -> ("Valve position (%)"=w295:dbl, "read pressure"=w289:dbl, "read vapor flow"=w294:dbl, "read gas flow"=w293:dbl)
        n133 = case shown="True" w276 {
          tunnel: w274 -> [_ w427]
          frame False {
          }
          frame True {
            n134 = Unbundle(w427) -> ("mean"=w426:dbl, "mean"=w425:dbl, "mean"=w424:dbl, "mean"=w423:dbl, "mean"=w422:dbl, "mean"=w420:dbl)
            n135 = Bundle("mean"=w426, "mean"=w426, "mean"=w425, "mean"=w425, "mean"=w424, "mean"=w424, "mean"=w423, "mean"=w423, "mean"=w422, "mean"=w422, "mean"=w420, "mean"=w420) -> (→"ArduinoQCM\ncluster":T36)  [unwired: 1 in]
          }
        }
        n136 = Unbundle("Data logging settings") -> ("Save during sequence only"=w374:bool, "Save now"=w376:bool, "sec between data points"=w363:dbl, "Save sample names"=w317:T37, "Experiment Notes"=w316:string)  [unwired: 1 out]
        n137 = property on="Valve position (%)" class="DigNum (strict)"("Value"=w295) -> ()  [unwired: 2 in, 2 out]
        n138 = Subtract(x=w361, y=w342) -> (x-y=w360:dbl)
        n139 = property on="read pressure" class="DigNum (strict)"("Value"=w289) -> ()  [unwired: 2 in, 2 out]
        n140 = And(x=w296, y=w374) -> (x .and. y?=w373:bool)
        n141 = Bundle("read pressure"=w289) -> (w288:cluster{"read pressure":dbl})  [unwired: 1 in]
        n142 = Divide(x=w360, y=60.0) -> (x/y=w334:dbl)
        "Elapsed time (min)" <- w334
        n143 = call "data_headers_subVI.vi"("Experiment Notes"=w316, "Sample names"=w317) -> ("data headers"=w387:string[])  [unwired: 9 in]
        n144 = property on="read vapor flow" class="DigNum (strict)"("Value"=w294) -> ()  [unwired: 2 in, 2 out]
        n145 = Multiply(x=w363, y=u32 1000 ("x")) -> (x*y=w396:dbl)
        n146 = Or(x=w373, y=w376) -> (x .or. y?=w370:bool)
        "saving data?" <- w370
        n147 = Wait (ms)(milliseconds to wait=w396) -> ()  [unwired: 1 out]
        n148 = property on="read gas flow" class="DigNum (strict)"("Value"=w293) -> ()  [unwired: 2 in, 2 out]
        n149 = property on="pressure chart" class="WFChart (strict)"("Value"=w288) -> ()  [unwired: 2 in, 2 out]
        n150 = Get Date/Time In Seconds() -> (seconds since 1Jan1904=w418:timestamp)
        n151 = Number To Engineering String ("elapsed time (min)")(4:w334) -> (0:w339:string)  [unwired: 3 in]
        n152 = Unbundle(w311) -> ("current  step # in"=w285:i32, "sequence end time in"=w310:timestamp, "Boolean"=w309:bool)
        n153 = Format Date/Time String(time format string (%c)="%Y-%m-%d %H:%M:%S%2u", seconds (now)=w418) -> (date/time string=w393:string)  [unwired: 1 in]
        n154 = Unbundle(w347) -> ("String data out"=w338:string, w337:string, w336:string, w335:string)
        n155 = Unbundle(w392) -> ("String"=w340:string, "String"=w395:string, "String"=w394:string)
        n156 = Unbundle(w331) -> ("String"=w330:string, "String"=w329:string)
        n157 = Unbundle(w298) -> ("pressure"=w386:string, "RH"=w385:string, "gas flow"=w384:string, "vapor flow"=w383:string)
        n158 = Unbundle ("arduino 1-6")(w279) -> ("mean"=w283:string, "mean"=w391:string, "mean"=w390:string, "mean"=w389:string, "mean"=w388:string, "mean"=w281:string)
        n159 = Increment(x=w285) -> (x+1=w284:i32)
        n160 = Build Array(w393, w339, w338, w337, w336, w335, w340, w395, w394, w330, w329, w386, w385, w384, w383, w282, w283, w391, w390, w389, w388, w281) -> (w401:string[])
        n161 = property on="Current\nstep" class="DigNum (strict)"("Value"=w284) -> ()  [unwired: 2 in, 2 out]
        "State date/time" <- w333
      }
      n162 = Unbundle(w85) -> (w84:bool, "VISA resource name out"=w83:refnum<visa-resource-name>, "error out"=w82:errorcluster)
      n163 = Unbundle(w81) -> ("Boolean"=w80:bool, "VISA out"=w79:refnum<visa-resource-name>, "error out"=w78:errorcluster)
      n164 = call-poly <vilib>:"Write To Spreadsheet File.vi"("1D data"=w49, "file path (dialog if empty)"=w66) -> ("new file path (Not A Path if cancelled)"=w70:path)  [unwired: 6 in]
      n165 = Unbundle(w59) -> (w64:bool, "VISA resource name out"=w63:refnum<visa-resource-name>, "error out"=w62:errorcluster)
      n166 = Unbundle(w27) -> ("Boolean"=w26:bool, "DAQ IDs in"=w25:T38)
      n167 = call "arduino_close_subIV.vi"("arduino 1-6 addresses and errors out"=w51, "arduinos on?"=w50) -> ()  [unwired: 10 in]
      n168 = case shown="True" w42 {
        tunnel: w41 -> [_ w100]
        tunnel: w40 -> [w97 w99]
        tunnel: [w97 w98] -> w39
        frame False {
        }
        frame True {
          n169 = call "Close.vi"("VISA resource name"=w100, "error in (no error)"=w99) -> ("error out"=w98:errorcluster)  [unwired: 17 in]
        }
      }
      n170 = flat-sequence {
        tunnel: w5 -> [w96]
        tunnel: [w96] -> w4
        frame #0 {
          n171 = property on="saving data?" class="Bool (strict)"("Value"=FALSE ("saving data?")) -> ()  [unwired: 2 in, 2 out]
        }
      }
      n172 = Unbundle(w76) -> ("Boolean"=w75:bool, "VISA resource name out"=w74:refnum<visa-resource-name>, "error out"=w73:errorcluster)
      n173 = case shown="True" w26 {
        tunnel: w25 -> [_ w128]
        tunnel: [errorcluster {"status"=FALSE, "code"=0, "source"=""} ("error out") w115] -> w34
        frame False {
        }
        frame True {
          n174 = Unbundle(w128) -> ("task out"=w127:refnum<k21>, "error out"=w126:errorcluster, "task out"=w125:refnum<k21>, "error out"=w124:errorcluster, "task out"=w123:refnum<k21>, "error out"=w122:errorcluster, "VISA Refnum out"=w121:refnum<visa-resource-name>, "error out"=w120:errorcluster)
          n175 = disable-structure shown="Disabled" {
            disable-tunnel: [w137 _] -> w119
            disable-tunnel: w127 -> [w136 _]
            disable-tunnel: w126 -> [w135 _]
            frame Disabled {
              n176 = call <vilib>:"DAQmx Stop Task.vi"("task/channels in"=w136, "error in"=w135) -> ("task out"=w138:refnum<k21>, "error out"=w139:errorcluster)  [unwired: 12 in]
              n177 = call <vilib>:"DAQmx Clear Task.vi"("task in"=w138, "error in"=w139) -> ("error out"=w137:errorcluster)  [unwired: 13 in]
            }
            frame Enabled {
            }
          }
          n178 = call <vilib>:"DAQmx Stop Task.vi"("task/channels in"=w125, "error in"=w124) -> ("task out"=w132:refnum<k21>, "error out"=w131:errorcluster)  [unwired: 12 in]
          n179 = call <vilib>:"DAQmx Stop Task.vi"("task/channels in"=w123, "error in"=w122) -> ("task out"=w133:refnum<k21>, "error out"=w134:errorcluster)  [unwired: 12 in]
          n180 = VISA Clear(VISA resource name=w121, error in (no error)=w120) -> (VISA resource name out=w130:refnum<visa-resource-name>, error out=w129:errorcluster)
          n181 = VISA Close(VISA resource name=w130, error in (no error)=w129) -> (error out=w116:errorcluster)
          n182 = call <vilib>:"DAQmx Clear Task.vi"("task in"=w132, "error in"=w131) -> ("error out"=w118:errorcluster)  [unwired: 13 in]
          n183 = call <vilib>:"DAQmx Clear Task.vi"("task in"=w133, "error in"=w134) -> ("error out"=w117:errorcluster)  [unwired: 13 in]
          n184 = Merge Errors(w119, w118, w117, w116) -> (w115:errorcluster)
        }
      }
      n185 = case shown="True" w84 {
        tunnel: w83 -> [_ w248]
        tunnel: w82 -> [w245 w247]
        tunnel: [w245 w246] -> w86
        frame False {
        }
        frame True {
          n186 = call "Enable Output.vi"("error in (no error)"=w247, "Enable Output (T: Enable)"=FALSE, "VISA resource name"=w248) -> ("error out"=w249:errorcluster, "VISA resource name out"=w251:refnum<visa-resource-name>)  [unwired: 7 in]
          n187 = call "Close.vi"("error in (no error)"=w249, "VISA resource name"=w251) -> ("error out"=w246:errorcluster)  [unwired: 9 in]
        }
      }
      n188 = case shown="True" w64 {
        tunnel: w63 -> [_ w163]
        tunnel: w62 -> [w161 w162]
        tunnel: [w161 w164] -> w58
        frame False {
        }
        frame True {
          n189 = call "Enable Output.vi"("error in (no error)"=w162, "Enable Output (F:Off)"=FALSE ("Output (F:Off)"), "VISA resource name"=w163) -> ("error out"=w165:errorcluster, "VISA resource name out"=w166:refnum<visa-resource-name>)  [unwired: 7 out]
          n190 = call "Close.vi"("error in (no error)"=w165, "VISA resource name"=w166) -> ("error out"=w164:errorcluster)  [unwired: 9 out]
        }
      }
      n191 = case shown="True" w80 {
        tunnel: w78 -> [w231 w234]
        tunnel: [w231 w233] -> w87
        tunnel: w79 -> [_ w232]
        frame False {
        }
        frame True {
          n192 = call "srsQcm200Close.vi"("error in"=w234, "Visa in"=w232) -> ("error out"=w233:errorcluster)  [unwired: 3 in]
        }
      }
      n193 = call-poly <vilib>:"Write To Spreadsheet File.vi"("append to file? (new file:F)"=TRUE, "2D data"=w53, "file path (dialog if empty)"=w70) -> ()  [unwired: 5 in, 1 out]
      n194 = case shown="True" w75 {
        tunnel: w74 -> [_ w201]
        tunnel: w73 -> [w198 w200]
        tunnel: [w198 w199] -> w72
        frame False {
        }
        frame True {
          n195 = VISA Close(VISA resource name=w201, error in (no error)=w200) -> (error out=w199:errorcluster)
        }
      }
      n196 = Merge Errors(w58, w72, w86, w39, w87, w4) -> (w93:errorcluster)
      n197 = call <vilib>:"Simple Error Handler.vi"("error in (no error)"=w34) -> ()  [unwired: 4 in, 5 out]
      n198 = call <vilib>:"Simple Error Handler.vi"("error in (no error)"=w93) -> ()  [unwired: 4 in, 5 out]
    }
  }
